vi "sum_regs.vi"(0 "Register Values":dbl[](array[numeric]), 2 "Old Time":u32) -> (1 "New Time":u32, 3 "Old Volume":dbl, 4 "dV Sum":dbl, 5 "dt Sum":dbl, 6 "Time diff (s)":dbl)   [LabVIEW 2015]
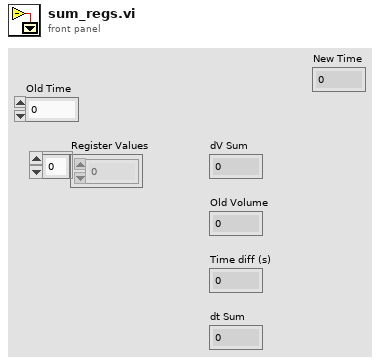
[diagram p1: front panel]
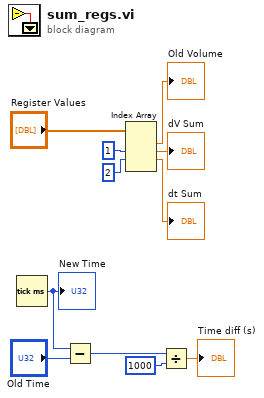
[diagram p0: block diagram]
diagram:
  n1 = Tick Count (ms)() -> (millisecond timer value=w5:u32)
  "New Time" <- w5
  n2 = Subtract(x=w5, y="Old Time") -> (x-y=w7:u32)
  n3 = Index Array(array="Register Values", index #2=1 ("index"), index #3=2 ("index")) -> (element #1=→"Old Volume":dbl, element #2=→"dV Sum":dbl, element #3=→"dt Sum":dbl)  [unwired: 2 in, 1 out]
  n4 = Divide(x=w7, y=u32 1000 ("x")) -> (x/y=→"Time diff (s)":dbl)
